vi "Map GD Errors.vi"(8 "error in (no error)":errorcluster caption="Fehler (Eingang, kein Fehler)", 9 "Störung Gasteiler":bool, 10 "Error":T2, 11 "Störung Kommunikation":bool) -> (0 "error out":errorcluster caption="Fehler (Ausgang)", 3 "LIN Errors-Cluster (Ausgang)":T1)   [LabVIEW 2020, in "Linearisierung v2.lvlib" / "Gasteiler.lvlib"]
uses:
  Gasteiler.lvlib
  Gasteiler Fehler.ctl
  LIN ErrorCluster.ctl
  Linearisierung v2.lvlib
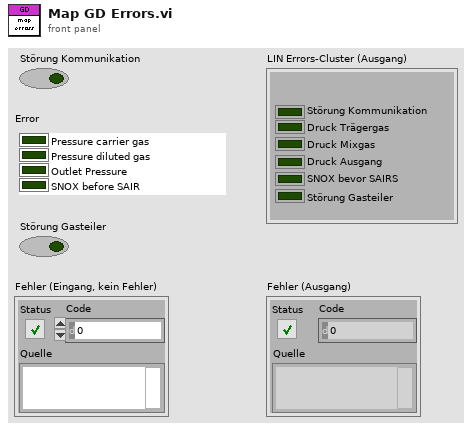
[diagram p1: front panel]
types:
  T1 = typedef "Linearisierung v2.lvlib/LIN ErrorCluster.ctl" = cluster{"Störung Kommunikation":bool, "Pressure carrier gas":bool, "Pressure diluted gas":bool, "Outlet Pressure":bool, "SNOX before SAIR":bool, "Störung Gasteiler":bool}
  T2 = typedef "Linearisierung v2.lvlib/Gasteiler.lvlib/Gasteiler Fehler.ctl" = cluster{"Pressure carrier gas":bool, "Pressure diluted gas":bool, "Outlet Pressure":bool, "SNOX before SAIR":bool}
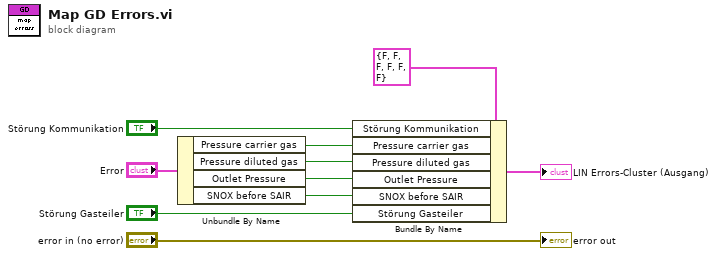
[diagram p0: block diagram]
diagram:
  n1 = Unbundle By Name("Error") -> ("Pressure carrier gas"=w10:bool, "Pressure diluted gas"=w3:bool, "Outlet Pressure"=w2:bool, "SNOX before SAIR"=w1:bool)
  n2 = Bundle By Name(cluster=T1 {"Störung Kommunikation"=FALSE, "Pressure carrier gas"=FALSE, "Pressure diluted gas"=FALSE, "Outlet Pressure"=FALSE, "SNOX before SAIR"=FALSE, "Störung Gasteiler"=FALSE} ("Ausgangs-Cluster"), "Störung Kommunikation"="Störung Kommunikation", "Pressure carrier gas"=w10, "Pressure diluted gas"=w3, "Outlet Pressure"=w2, "SNOX before SAIR"=w1, "Störung Gasteiler"="Störung Gasteiler") -> (→"LIN Errors-Cluster (Ausgang)":T1)
  "error out" <- "error in (no error)"
